vi "数据保存.vi"(4 "error in (no error)":errorcluster, 5 "数据库引用输入":T1, 6 "数据库文件名":string, 7 "队列":refnum<queue>) -> (1 "error out":errorcluster, 2 "队列引用输出":refnum<queue>, 3 "数据库引用输出":T1)   [LabVIEW 2014]
uses:
  <vilib>/addons/database/Connection.llb/Conn ObjectReference.ctl
  <vilib>/addons/database/NI_Database_API.lvlib
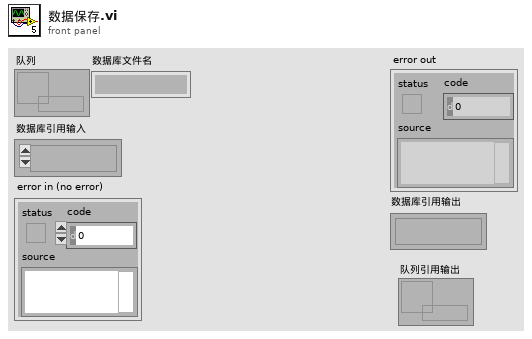
[diagram p1: front panel]
types:
  T1 = typedef "NI_Database_API.lvlib/Conn ObjectReference.ctl" = refnum<k1>
  T2 = cluster{i32, i32, i32, i32, i32, i32, i32, i32, i32, i32, i32, i32, string}
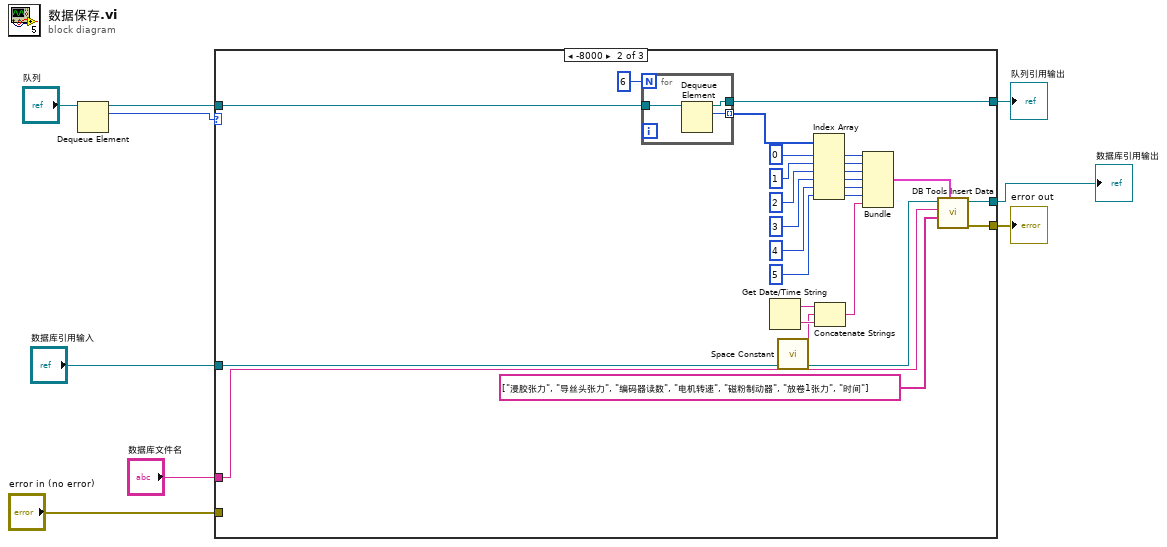
[diagram p0: block diagram]
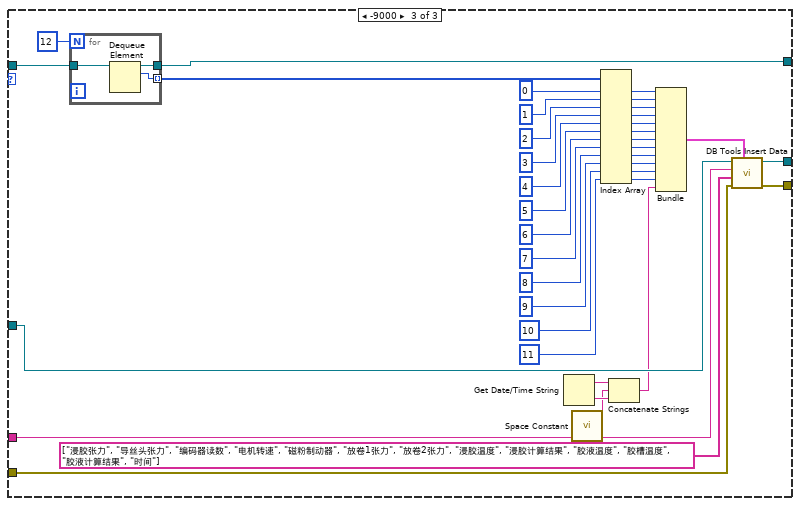
[diagram p3: hidden frame]
diagram:
  n1 = Dequeue Element(queue="队列") -> (queue out=w7:refnum<queue>, element=w8:i32)  [unwired: 2 in, 2 out]
  n2 = case shown="-8000" w8 {
    tunnel: w7 -> [w10 w38 w67]
    tunnel: "数据库文件名" -> [_ w26 w66]
    tunnel: "数据库引用输入" -> [w11 w25 w65]
    tunnel: "error in (no error)" -> [w12 _ w47]
    tunnel: [w12 w24 w46] -> w3
    tunnel: [w11 w23 w45] -> w2
    tunnel: [w10 w22 w44] -> w1
    frame 0, Default {
    }
    frame -8000 {
      n3 = for {
        N: 6 -> [_]
        tunnel: w38 -> [w41]
        tunnel: [w40] -> w36 mode=indexing
        tunnel: [w39] -> w22
        n4 = Dequeue Element(queue=w41) -> (queue out=w39:refnum<queue>, element=w40:i32)  [unwired: 2 in, 2 out]
      }
      n5 = Get Date/Time String ("获取日期/时间字符串")() -> (date string=w32:string, time string=w31:string)  [unwired: 3 in]
      n6 = call <vilib>:"Space Constant.vi"() -> ("String"=w20:string)
      n7 = Index Array(array=w36, index #1=0 ("索引"), index #2=1 ("索引"), index #3=2 ("索引"), index #4=3 ("索引"), index #5=4 ("索引"), index #6=5 ("索引")) -> (element #1=w30:i32, element #2=w29:i32, element #3=w28:i32, element #4=w16:i32, element #5=w15:i32, element #6=w14:i32)
      n8 = Concatenate Strings(w32, w20, w31) -> (w13:string)
      n9 = Bundle(w30, w29, w28, w16, w15, w14, w13) -> (w27:cluster{i32, i32, i32, i32, i32, i32, string})  [unwired: 1 in]
      n10 = call <vilib>:"DB Tools Insert Data.vi"("data"=w27, "columns"=string[] ["浸胶张力", "导丝头张力", "编码器读数", "电机转速", "磁粉制动器", "放卷1张力", "时间"], "table"=w26, "connection reference"=w25) -> ("error out"=w24:errorcluster, "connection reference out"=w23:T1)  [unwired: 6 in]
    }
    frame -9000 {
      n11 = for {
        N: 12 -> [_]
        tunnel: w67 -> [w83]
        tunnel: [w82] -> w79 mode=indexing
        tunnel: [w81] -> w44
        n12 = Dequeue Element(queue=w83) -> (queue out=w81:refnum<queue>, element=w82:i32)  [unwired: 2 in, 2 out]
      }
      n13 = Get Date/Time String ("获取日期/时间字符串")() -> (date string=w74:string, time string=w73:string)  [unwired: 3 in]
      n14 = call <vilib>:"Space Constant.vi"() -> ("String"=w72:string)
      n15 = Index Array(array=w79, index #1=0 ("索引"), index #2=1 ("索引"), index #3=2 ("索引"), index #4=3 ("索引"), index #5=4 ("索引"), index #6=5 ("索引"), index #7=6 ("索引"), index #8=7 ("索引"), index #9=8 ("索引"), index #10=9 ("索引"), index #11=10 ("索引"), index #12=11 ("索引")) -> (element #1=w71:i32, element #2=w70:i32, element #3=w69:i32, element #4=w68:i32, element #5=w56:i32, element #6=w55:i32, element #7=w54:i32, element #8=w53:i32, element #9=w52:i32, element #10=w51:i32, element #11=w50:i32, element #12=w49:i32)
      n16 = Concatenate Strings(w74, w72, w73) -> (w43:string)
      n17 = Bundle(w71, w70, w69, w68, w56, w55, w54, w53, w52, w51, w50, w49, w43) -> (w48:T2)  [unwired: 1 in]
      n18 = call <vilib>:"DB Tools Insert Data.vi"("data"=w48, "error in (no error)"=w47, "columns"=string[] ["浸胶张力", "导丝头张力", "编码器读数", "电机转速", "磁粉制动器", "放卷1张力", "放卷2张力", "浸胶温度", "浸胶计算结果", "胶液温度", "胶槽温度", "胶液计算结果", "时间"], "table"=w66, "connection reference"=w65) -> ("error out"=w46:errorcluster, "connection reference out"=w45:T1)  [unwired: 5 in]
    }
  }
  "数据库引用输出" <- w2
  "error out" <- w3
  "队列引用输出" <- w1
